vi "whatsVisibleU.vi"(11 "UplotInfoArray":T1(array[cluster])) -> (1 "Targets Visible":bool[](array[boolean]), 2 "Fits Visible":bool[](array[boolean]), 3 "BasicsVisible":bool[](array[boolean]))   [LabVIEW 2014]
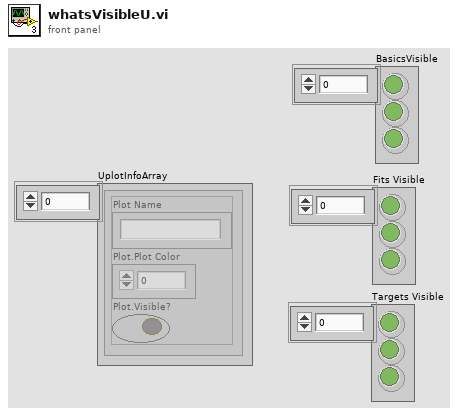
[diagram p1: front panel]
types:
  T1 = cluster{"Plot Name":string, "Plot.Plot Color":u32, "Plot.Visible?":bool}[]
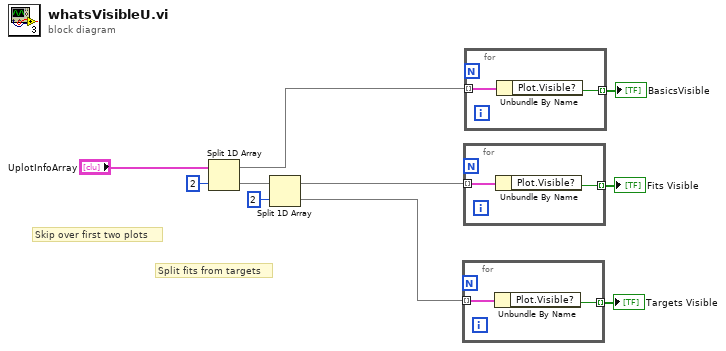
[diagram p0: block diagram]
diagram:
  # "Split fits from targets"
  # "Skip over first two plots"
  n1 = Split 1D Array(array="UplotInfoArray", index=2) -> (first subarray=w1:T1, second subarray=w8:T1)
  n2 = Split 1D Array(array=w8, index=2) -> (first subarray=w6:T1, second subarray=w3:T1)
  n3 = for {
    tunnel: w3 -> [w12] mode=indexing
    tunnel: [w11] -> w4 mode=indexing
    n4 = Unbundle By Name(w12) -> ("Plot.Visible?"=w11:bool)
  }
  "Targets Visible" <- w4
  n5 = for {
    tunnel: w6 -> [w14] mode=indexing
    tunnel: [w13] -> w5 mode=indexing
    n6 = Unbundle By Name(w14) -> ("Plot.Visible?"=w13:bool)
  }
  "Fits Visible" <- w5
  n7 = for {
    tunnel: w1 -> [w16] mode=indexing
    tunnel: [w15] -> w2 mode=indexing
    n8 = Unbundle By Name(w16) -> ("Plot.Visible?"=w15:bool)
  }
  "BasicsVisible" <- w2
